vi "drawBlacks.vi"(1 "Array 2":cluster{"Numeric":dbl, "Numeric 2":dbl}[](array[cluster]), 2 "Array 3":bool[][](array[boolean])) -> (0 "Array":bool[][](array[boolean]))   [LabVIEW 2009]
uses:
  Global 3.vi
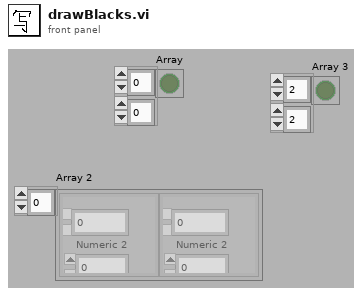
[diagram p1: front panel]
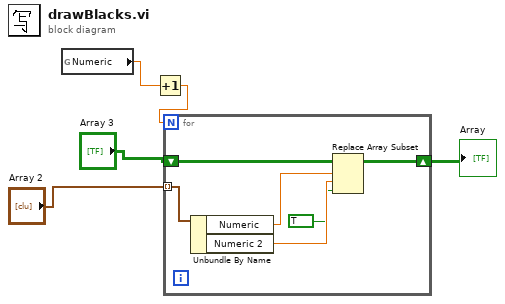
[diagram p0: block diagram]
diagram:
  n1 = global read "Global 3.vi" "Numeric"() -> (w5:dbl)
  n2 = Increment(x=w5) -> (x+1=w4:dbl)
  n3 = for {
    N: w4 -> [_]
    shift-right: [w11] -> w2
    shift-left: "Array 3" -> [w10]
    tunnel: "Array 2" -> [w6] mode=indexing
    n4 = Unbundle By Name(w6) -> ("Numeric"=w9:dbl, "Numeric 2"=w8:dbl)
    n5 = Replace Array Subset(array=w10, new element=TRUE ("new element/subarray"), index (row)=w9, index (col)=w8) -> (w11:bool[][])
  }
  "Array" <- w2
